vi "XML_Parse.vi"(8 "error in (no error)":errorcluster caption="错误输入（无错误）", 10 "Tag":string="opcua_server", 11 "XML":string="<opcua_server><name>server</name><port>4845</port><policy>none</policy><serverCertification></serverCertification><trustedClientCertifications><certification></certification></trustedClientCertifications><structure><folder name=\"all supported datatypes\"><folder name=\"singal element\"><item name=\"boolean\" access=\"read/write\" datatype=\"boolean\" initialValue=\"TRUE\"></item><item name=\"string\" access=\"read/write\" datatype=\"string\" initialValue=\"stringtype\"></item><item name=\"sbyte\" access=\"read/write\" datatype=\"sbyte\" initialValue=\"-10\"></item><item name=\"byte\" access=\"read/write\" datatype=\"byte\" initialValue=\"10\"></item><item name=\"int16\" access=\"read/write\" datatype=\"int16\" initialValue=\"-10\"></item><item name=\"int32\" access=\"read/write\" datatype=\"int32\" initialValue=\"-20\"></item><item name=\"int64\" access=\"read/write\" datatype=\"int64\" initialValue=\"-30\"></item><item name=\"uint16\" access=\"read/write\" datatype=\"uint16\" initialValue=\"10\"></item><item name=\"uint32\" access=\"read/write\" datatype=\"uint32\" initialValue=\"20\"></item><item name=\"uint64\" access=\"read/write\" datatype=\"uint64\" initialValue=\"30\"></item><item name=\"double\" access=\"read/write\" datatype=\"double\" initialValue=\"10.1\"></item><item name=\"float\" access=\"read/write\" datatype=\"float\" initialValue=\"12.1\"></item><item name=\"datetime\" access=\"read/write\" datatype=\"datetime\" initialValue=\"4/30/2004 7:48:47 PM\"></item><item name=\"byte string\" access=\"read/write\" datatype=\"ByteString\" initialValue=\"(1,2,3,4,5)\"></item></folder><folder name=\"array\"><item name=\"boolean array\" access=\"read/write\" datatype=\"boolean array\" initialValue=\"FALSE,TRUE,FALSE\"></item><item name=\"string array\" access=\"read/write\" datatype=\"string array\" initialValue=\"str1,str2,str3\"></item><item name=\"sbyte array\" access=\"read/write\" datatype=\"sbyte array\" initialValue=\"-1,2,-3,4,-5,6,-7,8\"></item><item name=\"byte array\" access=\"read/write\" datatype=\"byte array\" initialValue=\"1,2,3,4,5,6,7,8\"></item><item name=\"int16 array\" access=\"read/write\" datatype=\"int16 array\" initialValue=\"-1,2,-3,4,-5,6,-7,8\"></item><item name=\"int32 array\" access=\"read/write\" datatype=\"int32 array\" initialValue=\"-1,2,-3,4,-5,6,-7,8\"></item><item name=\"int64 array\" access=\"read/write\" datatype=\"int64 array\" initialValue=\"-1,2,-3,4,-5,6,-7,8\"></item><item name=\"uint16 array\" access=\"read/write\" datatype=\"uint16 array\" initialValue=\"1,2,3,4,5,6,7,8\"></item><item name=\"uint32 array\" access=\"read/write\" datatype=\"uint32 array\" initialValue=\"1,2,3,4,5,6,7,8\"></item><item name=\"uint64 array\" access=\"read/write\" datatype=\"uint64 array\" initialValue=\"1,2,3,4,5,6,7,8\"></item><item name=\"double array\" access=\"read/write\" datatype=\"double array\" initialValue=\"1.1,2.2,3.3\"></item><item name=\"float array\" access=\"read/write\" datatype=\"float array\" initialValue=\"1.1,2.2,3.3\"></item><item name=\"datetime array\" access=\"read/write\" datatype=\"datetime array\" initialValue=\"4/30/2004 7:48:47 PM,5/30/2004 8:48:47 PM,6/30/2004 9:48:47 PM\"></item></folder></folder><folder name=\"structure demo\"><folder name=\"device1\"><item name=\"int1\" access=\"read/write\" datatype=\"int32\" initialValue=\"50\" description=\"\"><property name=\"set point\" access=\"read/write\" datatype=\"int32\" initialValue=\"12.4\" description=\"Set point of int1.\"></property><property name=\"status\" access=\"read only\" datatype=\"boolean\" initialValue=\"FALSE\" description=\"Status of int1.\"></property></item></folder><folder name=\"device2\"><folder name=\"device3\"><item name=\"bool1\" access=\"read/write\" datatype=\"boolean\" initialValue=\"FALSE\" description=\"\"><property name=\"set point\" access=\"read/write\" datatype=\"boolean\" initialValue=\"FALSE\" description=\"Set point of bool1.\"></property><property name=\"status\" access=\"read only\" datatype=\"boolean\" initialValue=\"FALSE\" description=\"Status of bool1.\"></property></item></folder><item name=\"str1\" access=\"read/write\" datatype=\"string\" initialValue=\"\" description=\"\"><property name=\"set point\" access=\"read/write\" datatype=\"string\" initialValue=\"test initialize\" description=\"Set point of str1.\"></property><property name=\"status\" access=\"read only\" datatype=\"boolean\" initialValue=\"FALSE\" description=\"Status of str1.\"></property></item></folder><folder name=\"grandpa\"><folder name=\"father\"><folder name=\"son\"><item name=\"son item\" access=\"read/write\" datatype=\"string\" initialValue=\"\" description=\"\"></item></folder></folder></folder><folder name=\"level1\"><folder name=\"level2\"><folder name=\"level3\"><folder name=\"level4\"><folder name=\"level5\"><folder name=\"level6\"><item name=\"data level6\" access=\"read/write\" datatype=\"uint32\" initialValue=\"1000\" description=\"\"></item></folder></folder></folder></folder></folder></folder></folder></structure></opcua_server>") -> (0 "error out":errorcluster caption="错误输出", 1 "keyValues":cluster{"key":string, "value":string}[](array[cluster]), 2 "match substring":string, 3 "content":string, 5 "after substring":string, 7 "before substring":string)   [LabVIEW 2014]
uses:
  <userlib>/_OpenG.lib/string/string.llb/Trim Whitespace (String)__ogtk.vi
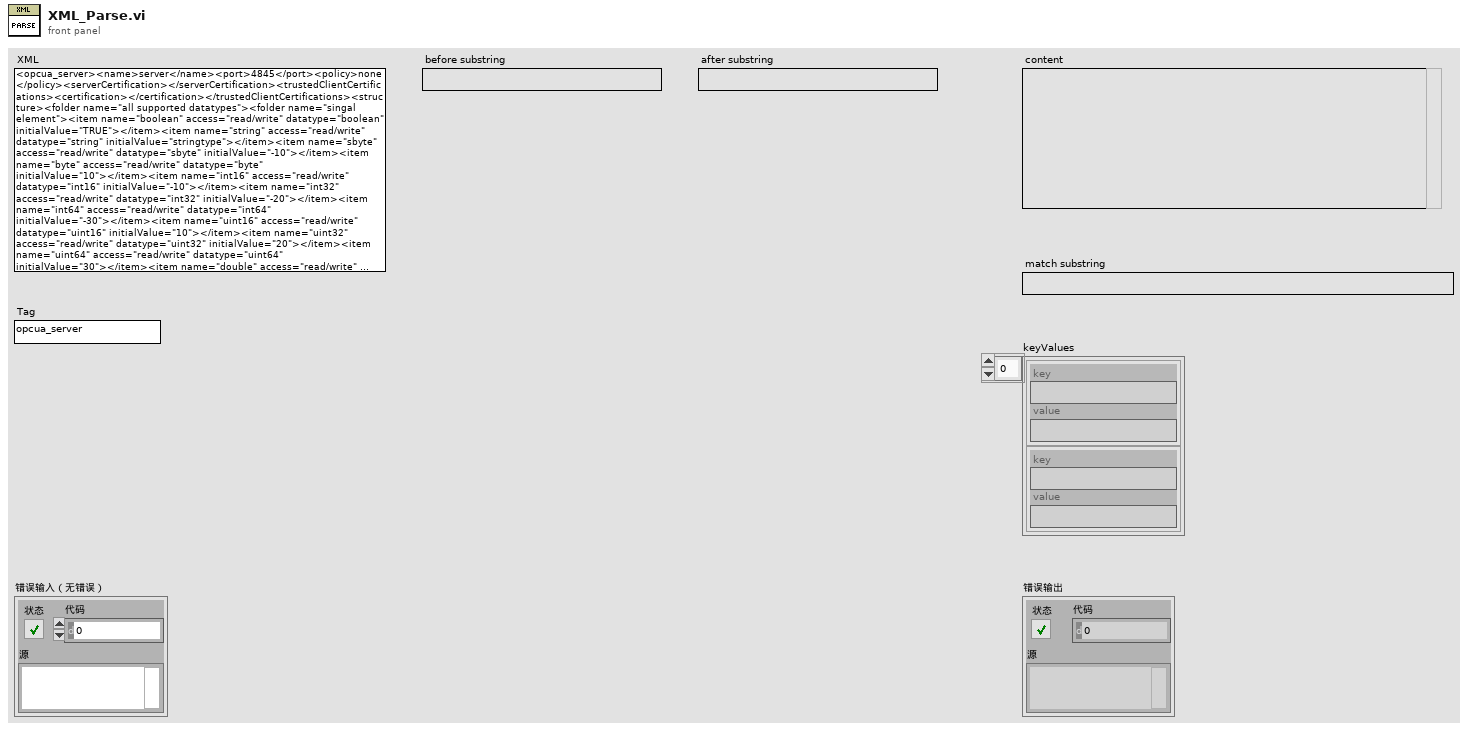
[diagram p1: front panel]
types:
  T1 = cluster{"whole match":string, "whole match":string}[]
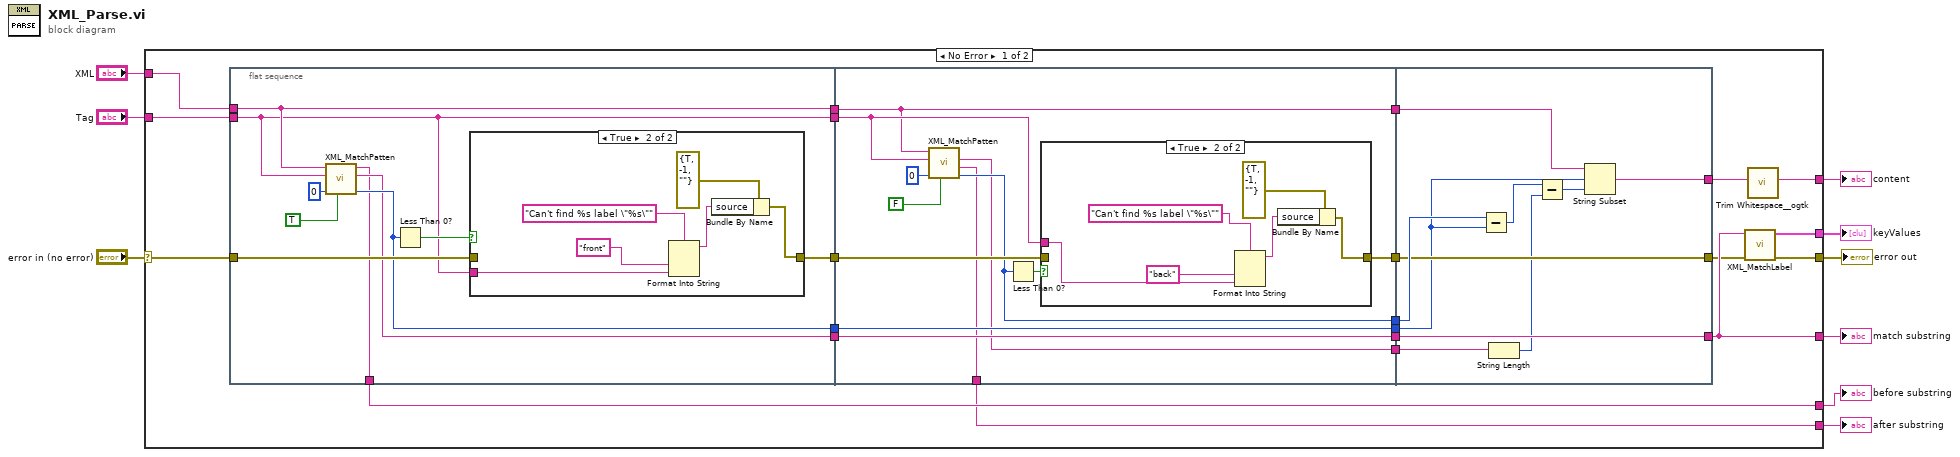
[diagram p0: block diagram]
diagram:
  n1 = case shown="No Error" "error in (no error)" {
    selector: "error in (no error)" -> [w29 w78]
    tunnel: [w12 w78] -> w8
    tunnel: "Tag" -> [w30 _]
    tunnel: "XML" -> [w31 _]
    tunnel: [w10 _] -> w5
    tunnel: [w17 _] -> w4
    tunnel: [w16 _] -> w3
    tunnel: [w14 _] -> w2
    tunnel: [w11 _] -> w1
    frame No Error {
      n2 = flat-sequence {
        tunnel: w31 -> [w37]
        tunnel: w30 -> [w32]
        tunnel: w29 -> [w39]
        tunnel: [w38] -> w28
        tunnel: [w32] -> w27
        tunnel: [w37] -> w26
        tunnel: [w36] -> w23
        tunnel: [w35] -> w21
        tunnel: [w33] -> w17
        tunnel: w28 -> [w58]
        tunnel: w27 -> [w52]
        tunnel: w26 -> [w49]
        tunnel: [w49] -> w25
        tunnel: [w57] -> w24
        tunnel: w23 -> [w57]
        tunnel: [w56] -> w22
        tunnel: w21 -> [w55]
        tunnel: [w55] -> w20
        tunnel: [w54] -> w19
        tunnel: [w51] -> w16
        tunnel: [w50] -> w15
        tunnel: w25 -> [w77]
        tunnel: w24 -> [w72]
        tunnel: w22 -> [w76]
        tunnel: w20 -> [w73]
        tunnel: [w75] -> w13
        tunnel: w19 -> [w75]
        tunnel: [w74] -> w18
        tunnel: [w73] -> w14
        tunnel: w15 -> [w70]
        frame #0 {
          n3 = call "XML_MatchPatten.vi"("first(T)/Last(F)"=TRUE, "offset (0)"=0, "tag"=w32, "XML"=w37) -> ("offset past match"=w36:i32, "concatenated string out"=w35:string, "before substring"=w33:string)  [unwired: 4 in, 1 out]
          n4 = Less Than 0?(x=w36) -> (x < 0?=w40:bool)
          n5 = case shown="True" w40 {
            tunnel: w39 -> [w42 _]
            tunnel: [w42 w47] -> w38
            tunnel: w32 -> [_ w44]
            frame False {
            }
            frame True {
              n6 = Format Into String(format string="Can't find %s label \"%s\"", "front" ("format string"), w44) -> (resulting string=w46:string)  [unwired: 2 in, 1 out]
              n7 = Bundle By Name(cluster=errorcluster {"status"=TRUE, "code"=-1, "source"=""} ("error IO"), "source"=w46) -> (w47:errorcluster)
            }
          }
        }
        frame #1 {
          n8 = call "XML_MatchPatten.vi"("first(T)/Last(F)"=FALSE, "offset (0)"=0, "tag"=w52, "XML"=w49) -> ("offset past match"=w56:i32, "after substring"=w51:string, "concatenated string out"=w50:string)  [unwired: 4 in, 1 out]
          n9 = Less Than 0?(x=w56) -> (x < 0?=w59:bool)
          n10 = case shown="True" w59 {
            tunnel: [w61 w66] -> w54
            tunnel: w52 -> [_ w63]
            tunnel: w58 -> [w61 _]
            frame False {
            }
            frame True {
              n11 = Format Into String(format string="Can't find %s label \"%s\"", "back" ("format string"), w63) -> (resulting string=w65:string)  [unwired: 2 in, 1 out]
              n12 = Bundle By Name(cluster=errorcluster {"status"=TRUE, "code"=-1, "source"=""} ("error IO"), "source"=w65) -> (w66:errorcluster)
            }
          }
        }
        frame #2 {
          n13 = Subtract(x=w76, y=w72) -> (x-y=w69:i32)
          n14 = String Length(string=w70) -> (length=w71:i32)
          n15 = Subtract(x=w69, y=w71) -> (x-y=w68:i32)
          n16 = String Subset(string=w77, offset (0)=w72, length (rest)=w68) -> (substring=w74:string)
        }
      }
      n17 = call "XML_MatchLabel.vi"("error in (no error)"=w13, "String"=w14) -> ("error out"=w12:errorcluster, "keyValues"=w11:T1)  [unwired: 8 in]
      n18 = call-poly <userlib>:"Trim Whitespace__ogtk.vi"("String in"=w18) -> ("String out"=w10:string)  [unwired: 6 in]
    }
    frame Error {
    }
  }
  "error out" <- w8
  "content" <- w5
  "match substring" <- w2
  "after substring" <- w3
  "before substring" <- w4
  "keyValues" <- w1
